vi "Descrizione prove manager.vi"() -> ()   [LabVIEW 2019]
uses:
  TypeDef/Descrizione prove.ctl
  Global percorso impostazioni.vi
panel:
  in  "ANNULLA":bool
  in  "SALVA":bool
  in  "DESCRIZIONE PROVE":T1
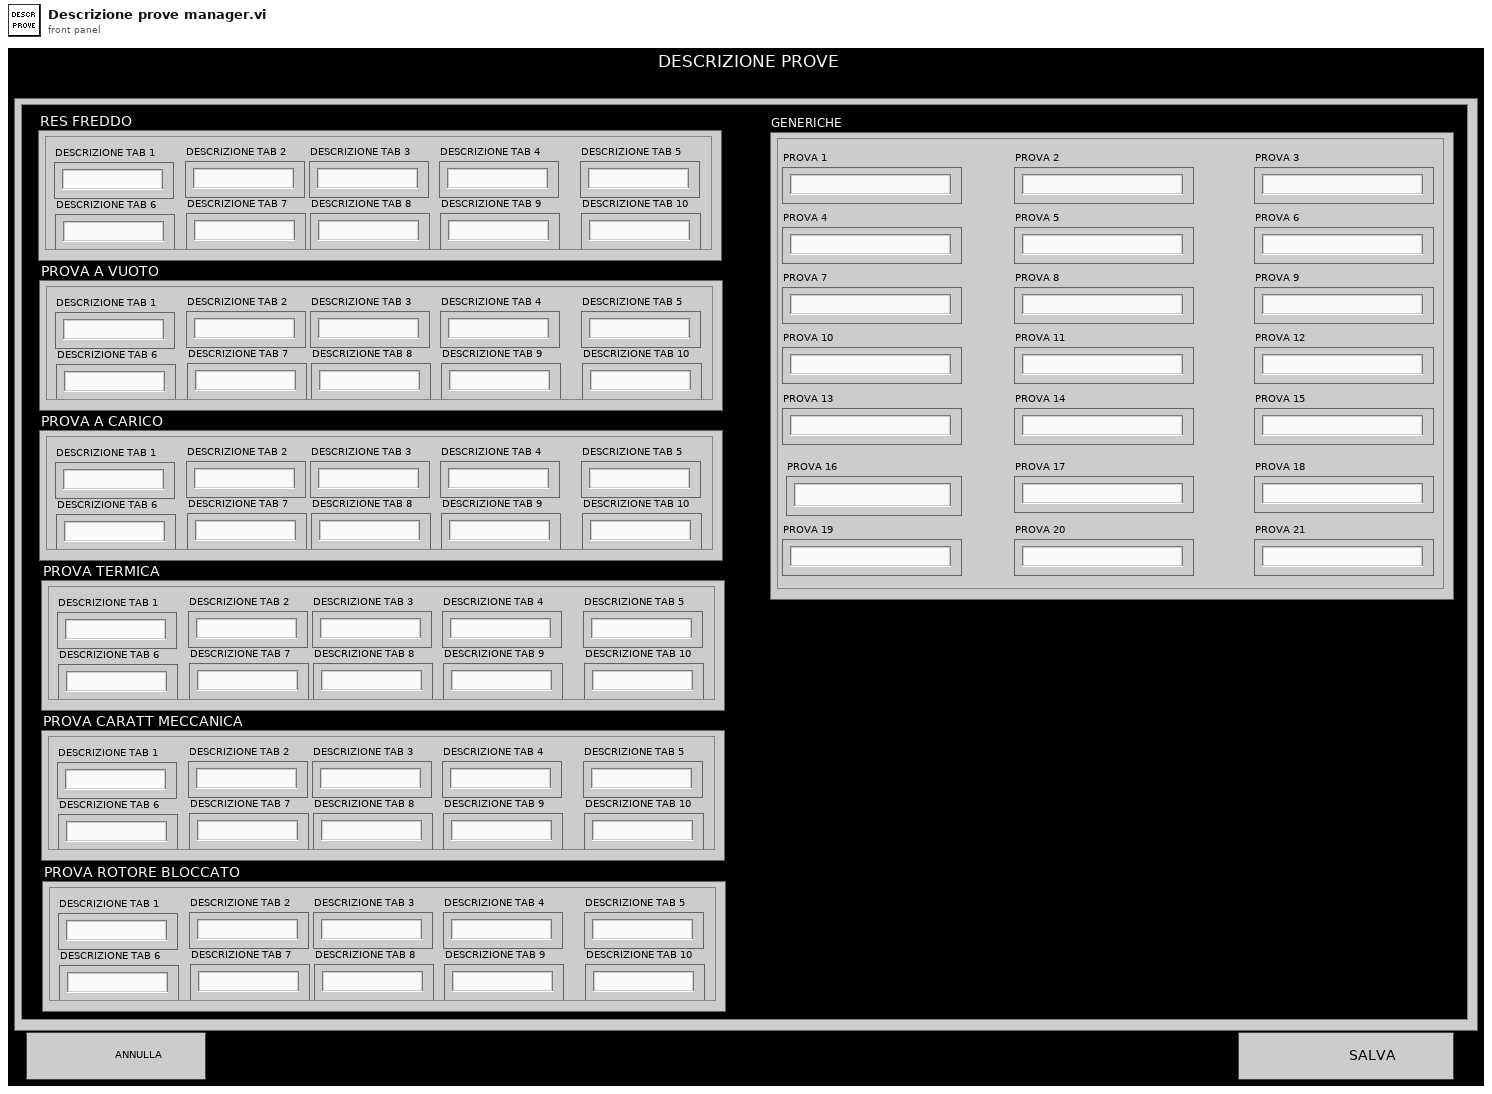
[diagram p1: front panel]
types:
  T1 = typedef "Descrizione prove.ctl" = cluster{"RES FREDDO":cluster{"DESCRIZIONE TAB 1":string, "DESCRIZIONE TAB 2":string, "DESCRIZIONE TAB 3":string, "DESCRIZIONE TAB 4":string, "DESCRIZIONE TAB 5":string, "DESCRIZIONE TAB 6":string, "DESCRIZIONE TAB 7":string, "DESCRIZIONE TAB 8":string, "DESCRIZIONE TAB 9":string, "DESCRIZIONE TAB 10":string}, "GENERICHE":cluster{"PROVA 1":string, "PROVA 2":string, "PROVA 3":string, "PROVA 4":string, "PROVA 5":string, "PROVA 6":string, "PROVA 7":string, "PROVA 8":string, "PROVA 9":string, "PROVA 10":string, "PROVA 11":string, "PROVA 12":string, "PROVA 13":string, "PROVA 14":string, "PROVA 15":string, "PROVA 16":string, "PROVA 17":string, "PROVA 18":string, "PROVA 19":string, "PROVA 20":string, "PROVA 21":string}, "PROVA A VUOTO":cluster{"DESCRIZIONE TAB 1":string, "DESCRIZIONE TAB 2":string, "DESCRIZIONE TAB 3":string, "DESCRIZIONE TAB 4":string, "DESCRIZIONE TAB 5":string, "DESCRIZIONE TAB 6":string, "DESCRIZIONE TAB 7":string, "DESCRIZIONE TAB 8":string, "DESCRIZIONE TAB 9":string, "DESCRIZIONE TAB 10":string}, "PROVA A CARICO":cluster{"DESCRIZIONE TAB 1":string, "DESCRIZIONE TAB 2":string, "DESCRIZIONE TAB 3":string, "DESCRIZIONE TAB 4":string, "DESCRIZIONE TAB 5":string, "DESCRIZIONE TAB 6":string, "DESCRIZIONE TAB 7":string, "DESCRIZIONE TAB 8":string, "DESCRIZIONE TAB 9":string, "DESCRIZIONE TAB 10":string}, "PROVA TERMICA":cluster{"DESCRIZIONE TAB 1":string, "DESCRIZIONE TAB 2":string, "DESCRIZIONE TAB 3":string, "DESCRIZIONE TAB 4":string, "DESCRIZIONE TAB 5":string, "DESCRIZIONE TAB 6":string, "DESCRIZIONE TAB 7":string, "DESCRIZIONE TAB 8":string, "DESCRIZIONE TAB 9":string, "DESCRIZIONE TAB 10":string}, "PROVA CARATT MECCANICA":cluster{"DESCRIZIONE TAB 1":string, "DESCRIZIONE TAB 2":string, "DESCRIZIONE TAB 3":string, "DESCRIZIONE TAB 4":string, "DESCRIZIONE TAB 5":string, "DESCRIZIONE TAB 6":string, "DESCRIZIONE TAB 7":string, "DESCRIZIONE TAB 8":string, "DESCRIZIONE TAB 9":string, "DESCRIZIONE TAB 10":string}, "PROVA ROTORE BLOCCATO":cluster{"DESCRIZIONE TAB 1":string, "DESCRIZIONE TAB 2":string, "DESCRIZIONE TAB 3":string, "DESCRIZIONE TAB 4":string, "DESCRIZIONE TAB 5":string, "DESCRIZIONE TAB 6":string, "DESCRIZIONE TAB 7":string, "DESCRIZIONE TAB 8":string, "DESCRIZIONE TAB 9":string, "DESCRIZIONE TAB 10":string}}
  T2 = enum16{"open", "replace", "create", "open or create", "replace or create", "replace or create with confirmation"}
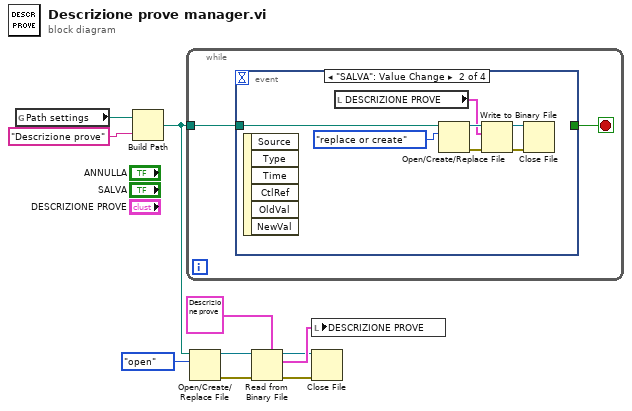
[diagram p0: block diagram]
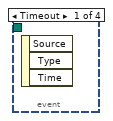
[diagram p2: hidden frame]
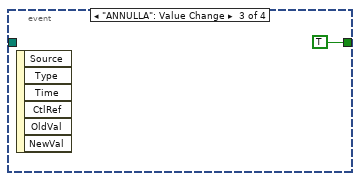
[diagram p3: hidden frame]
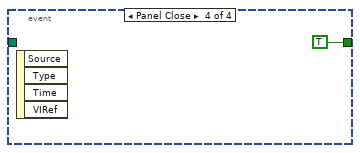
[diagram p4: hidden frame]
diagram:
  n1 = global read "Global percorso impostazioni.vi" "Path settings"() -> (w9:path)
  n2 = Build Path(base path=w9, name or relative path="Descrizione prove") -> (appended path=w1:path)
  n3 = while {
    tunnel: w1 -> [w11]
    stop <- w12 stop-if-true
    n4 = event shown="[1] \"SALVA\": Value Change" {
      selector: _ -> [_ _ _ _]
      dyn-events: _ -> [_ _ _ _]
      timeout: _ -> [_ _ _ _]
      tunnel: [_ _ TRUE TRUE] -> w12
      tunnel: w11 -> [_ w18 _ _]
      event Timeout {
        n5 = event-data() -> ()  [unwired: 1 in, 3 out]
      }
      event "SALVA": Value Change {
        n6 = event-data() -> ()  [unwired: 1 in, 6 out]
        n7 = local read "DESCRIZIONE PROVE"() -> (w15:T1)
        n8 = Open/Create/Replace File(file path (use dialog)=w18, operation (0:open)=T2."replace or create") -> (refnum out=w17:refnum<file>, error out=w16:errorcluster)  [unwired: 4 in, 1 out]
        n9 = Write to Binary File(file (use dialog)=w17, data=w15, error in=w16) -> (refnum out=w13:refnum<file>, error out=w14:errorcluster)  [unwired: 3 in, 1 out]
        n10 = Close File(refnum=w13, error in=w14) -> ()  [unwired: 2 out]
      }
      event "ANNULLA": Value Change {
        n11 = event-data() -> ()  [unwired: 1 in, 6 out]
      }
      event Panel Close {
        n12 = event-data() -> ()  [unwired: 1 in, 4 out]
      }
    }
  }
  n13 = Open/Create/Replace File(file path (use dialog)=w1, operation (0:open)=T2."open") -> (refnum out=w7:refnum<file>, error out=w6:errorcluster)  [unwired: 4 in, 1 out]
  n14 = Read from Binary File(5:T1 {"RES FREDDO"={"DESCRIZIONE TAB 1"="", "DESCRIZIONE TAB 2"="", "DESCRIZIONE TAB 3"="", "DESCRIZIONE TAB 4"="", "DESCRIZIONE TAB 5"="", "DESCRIZIONE TAB 6"="", "DESCRIZIONE TAB 7"="", "DESCRIZIONE TAB 8"="", "DESCRIZIONE TAB 9"="", "DESCRIZIONE TAB 10"=""}, "GENERICHE"={"PROVA 1"="", "PROVA 2"="", "PROVA 3"="", "PROVA 4"="", "PROVA 5"="", "PROVA 6"="", "PROVA 7"="", "PROVA 8"="", "PROVA 9"="", "PROVA 10"="", "PROVA 11"="", "PROVA 12"="", "PROVA 13"="", "PROVA 14"="", "PROVA 15"="", "PROVA 16"="", "PROVA 17"="", "PROVA 18"="", "PROVA 19"="", "PROVA 20"="", "PROVA 21"=""}, "PROVA A VUOTO"={"DESCRIZIONE TAB 1"="", "DESCRIZIONE TAB 2"="", "DESCRIZIONE TAB 3"="", "DESCRIZIONE TAB 4"="", "DESCRIZIONE TAB 5"="", "DESCRIZIONE TAB 6"="", "DESCRIZIONE TAB 7"="", "DESCRIZIONE TAB 8"="", "DESCRIZIONE TAB 9"="", "DESCRIZIONE TAB 10"=""}, "PROVA A CARICO"={"DESCRIZIONE TAB 1"="", "DESCRIZIONE TAB 2"="", "DESCRIZIONE TAB 3"="", "DESCRIZIONE TAB 4"="", "DESCRIZIONE TAB 5"="", "DESCRIZIONE TAB 6"="", "DESCRIZIONE TAB 7"="", "DESCRIZIONE TAB 8"="", "DESCRIZIONE TAB 9"="", "DESCRIZIONE TAB 10"=""}, "PROVA TERMICA"={"DESCRIZIONE TAB 1"="", "DESCRIZIONE TAB 2"="", "DESCRIZIONE TAB 3"="", "DESCRIZIONE TAB 4"="", "DESCRIZIONE TAB 5"="", "DESCRIZIONE TAB 6"="", "DESCRIZIONE TAB 7"="", "DESCRIZIONE TAB 8"="", "DESCRIZIONE TAB 9"="", "DESCRIZIONE TAB 10"=""}, "PROVA CARATT MECCANICA"={"DESCRIZIONE TAB 1"="", "DESCRIZIONE TAB 2"="", "DESCRIZIONE TAB 3"="", "DESCRIZIONE TAB 4"="", "DESCRIZIONE TAB 5"="", "DESCRIZIONE TAB 6"="", "DESCRIZIONE TAB 7"="", "DESCRIZIONE TAB 8"="", "DESCRIZIONE TAB 9"="", "DESCRIZIONE TAB 10"=""}, "PROVA ROTORE BLOCCATO"={"DESCRIZIONE TAB 1"="", "DESCRIZIONE TAB 2"="", "DESCRIZIONE TAB 3"="", "DESCRIZIONE TAB 4"="", "DESCRIZIONE TAB 5"="", "DESCRIZIONE TAB 6"="", "DESCRIZIONE TAB 7"="", "DESCRIZIONE TAB 8"="", "DESCRIZIONE TAB 9"="", "DESCRIZIONE TAB 10"=""}} ("DESCRIZIONE PROVE"), 8:w6, 11:w7) -> (0:w2:errorcluster, 2:w4:T1, 3:w3:refnum<file>)  [unwired: 3 in, 1 out]
  n15 = local write "DESCRIZIONE PROVE"(w4) -> ()
  n16 = Close File(refnum=w3, error in=w2) -> ()  [unwired: 2 out]
